vi "StrNumConv.vi"(2 "Freq. String":string) -> (6 "Freq.":dbl)   [LabVIEW 2018]
uses:
  <vilib>/regexp/Match Regular Expression.xnode
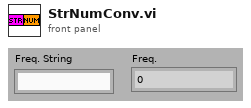
[diagram p1: front panel]
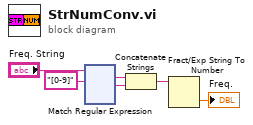
[diagram p0: block diagram]
diagram:
  n1 = xnode "Match Regular Expression"("input string"="Freq. String", "regular expression"="[0-9]") -> ("whole match"=w4:string, "after match"=w5:string)  [unwired: 4 in, 3 out]
  n2 = Concatenate Strings(w4, w5) -> (w6:string)
  n3 = Fract/Exp String To Number(string=w6) -> (number=→"Freq.":dbl)  [unwired: 3 in, 1 out]
